vi "Convert Node.vi"(6 "Mouse Position":T1, 7 "User VI Ref":refnum<vi>, 8 "Is Multi-select?":bool, 9 "Remaining Items":refnum<vi>[](array[refnum]), 10 "Affected Items":T8, 11 "Menu Refnum":refnum<k9>) -> (3 "Menu Items To Add":T2[](array[typedef]))   [LabVIEW 2020]
doc: "This VI is part of a plug-in for modifying the LabVIEW shortcut menus. This is the builder VI which is called when the shortcut menu is built. It tells LabVIEW which shortcut menu items to add to the menu."
uses:
  <resource>/plugins/PopupMenus/support/Shortcut Menu Item Definition.ctl
  <resource>/plugins/PopupMenus/support/Transaction Control.ctl
  <resource>/plugins/PopupMenus/support/Position In Menu.ctl
  <resource>/plugins/PopupMenus/support/Relative Position.ctl
  <resource>/plugins/PopupMenus/support/Checkmark Status.ctl
  <resource>/plugins/PopupMenus/support/Enabled Menu Item Status.ctl
  Convert Node.ctl
  <vilib>/Utility/miscctls.llb/LVPositionTypeDef.ctl
panel:
  # "Rules a popup plug-in must follow:\n* This VI's file name must match the file name of the LLB -- only the file extensions should be different.\n* This VI must have debugging disabled or it will be ignored as a plug-in.\n* For all menu items, \"tag suffix + file name of this VI\" must be less than 240 characters.\n* You can disconnect the \"Affected Items\" from the typedef to make the plug-in load faster. The typedef is only there to assist you in keeping this VI and the execution VI using to the same type.\n* All controls on this panel except \"Affected Items\" are locked to prevent accidental edits. Do not change the types or the names of controls other than the elements inside the \"Affected Items\" cluster.\n* See Context Help for more information on the individual controls."
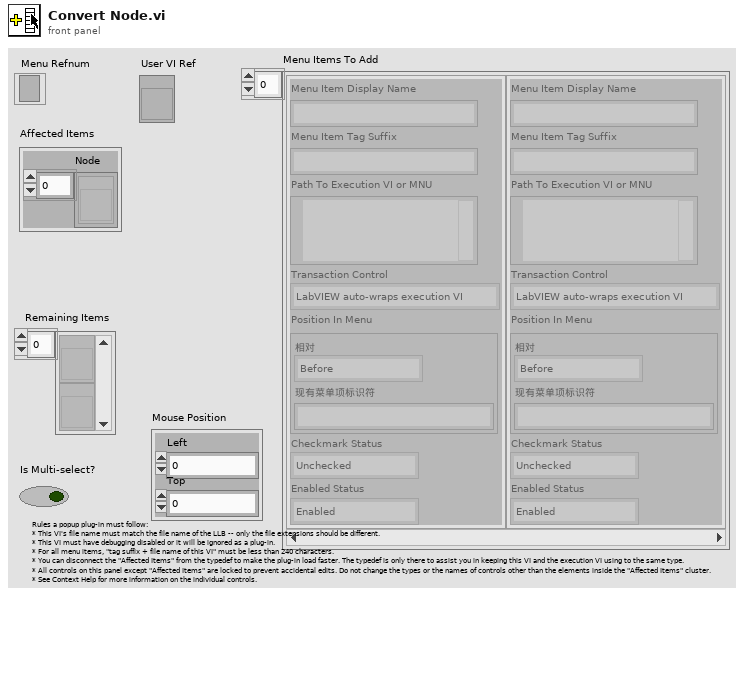
[diagram p1: front panel]
types:
  T1 = typedef "LVPositionTypeDef.ctl" = cluster{"Left":i32, "Top":i32}
  T2 = typedef "Shortcut Menu Item Definition.ctl" = cluster{"Menu Item Display Name":string, "Menu Item Tag Suffix":string, "Path To Execution VI or MNU":path, "Transaction Control":T3, "Position In Menu":T4, "Checkmark Status":T6, "Enabled Status":T7}
  T3 = typedef "Transaction Control.ctl" = enum8{"LabVIEW auto-wraps execution VI", "Execution VI will define if needed"}
  T4 = typedef "Position In Menu.ctl" = cluster{"Relative":T5, "Existing Item Tag":string}
  T5 = typedef "Relative Position.ctl" = enum8{"Before", "Instead of", "After", "Into Submenu"}
  T6 = typedef "Checkmark Status.ctl" = enum8{"Unchecked", "Checked"}
  T7 = typedef "Enabled Menu Item Status.ctl" = enum8{"Enabled", "Disabled"}
  T8 = typedef "Convert Node.ctl" = cluster{"Node":refnum<vi>[]}
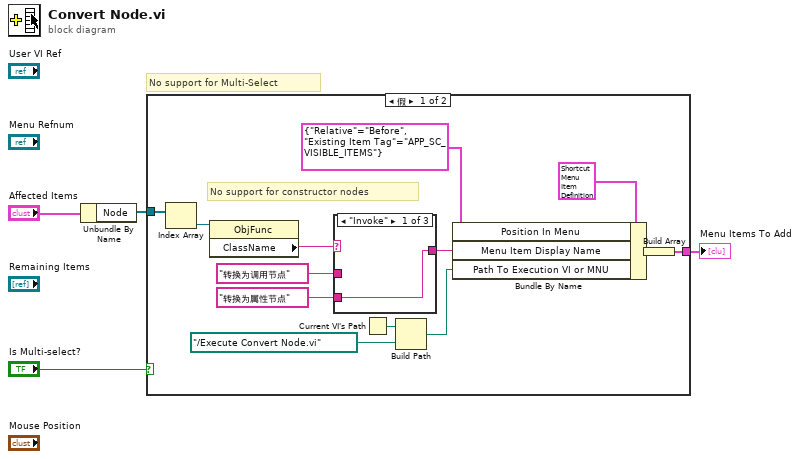
[diagram p0: block diagram]
diagram:
  # "No support for Multi-Select"
  n1 = Unbundle By Name("Affected Items") -> ("Node"=w2:refnum<vi>[])
  n2 = case shown="假" "Is Multi-select?" {
    tunnel: [w13 _] -> w4
    tunnel: w2 -> [w11 _]
    frame False {
      # "No support for constructor nodes"
      n3 = Index Array(array=w11) -> (element=w10:refnum<vi>)  [unwired: 1 in]
      n4 = property class="ObjFunc"(reference=w10) -> ("ClassName"=w8:string)  [unwired: 1 in, 2 out]
      n5 = case shown="\"Invoke\"" w8 {
        tunnel: [w18 w19 _] -> w7
        tunnel: "转换为调用节点" ("y") -> [_ w19 _]
        tunnel: "转换为属性节点" ("y") -> [w18 _ _]
        frame "Invoke" {
        }
        frame "Property" {
        }
        frame Default {
        }
      }
      n6 = Current VI's Path() -> (path=w12:path)
      n7 = Build Path(base path=w12, name or relative path=path "../Execute Convert Node.vi" ("execute path")) -> (appended path=w16:path)
      n8 = Bundle By Name(cluster=T2 {"Menu Item Display Name"="", "Menu Item Tag Suffix"="", "Path To Execution VI or MNU"=path "", "Transaction Control"=enum."LabVIEW auto-wraps execution VI", "Position In Menu"={"Relative"=enum."Before", "Existing Item Tag"=""}, "Checkmark Status"=enum."Unchecked", "Enabled Status"=enum."Enabled"} ("Cluster"), "Position In Menu"=T4 {"Relative"=enum."Before", "Existing Item Tag"="APP_SC_VISIBLE_ITEMS"}, "Menu Item Display Name"=w7, "Path To Execution VI or MNU"=w16) -> (w14:T2)
      n9 = Build Array(w14) -> (w13:T2[])
    }
    frame True {
    }
  }
  "Menu Items To Add" <- w4
